vi "De-construct.vi"(10 "msg o":string) -> (0 "MSES/SRES":string, 1 "RSP?":bool, 2 "Data":string, 5 "CMD":T1, 7 "header":string)   [LabVIEW 2020, in "FINS TCP.lvlib"]
uses:
  FINS TCP.lvlib
  FINS CMD.ctl
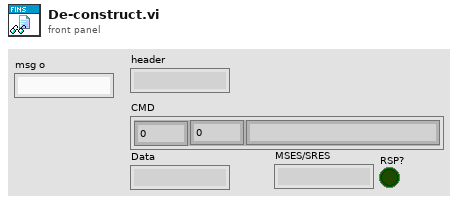
[diagram p1: front panel]
types:
  T1 = typedef "FINS TCP.lvlib/FINS CMD.ctl" = cluster{"MR":u8, "SR":u8, "name":string}
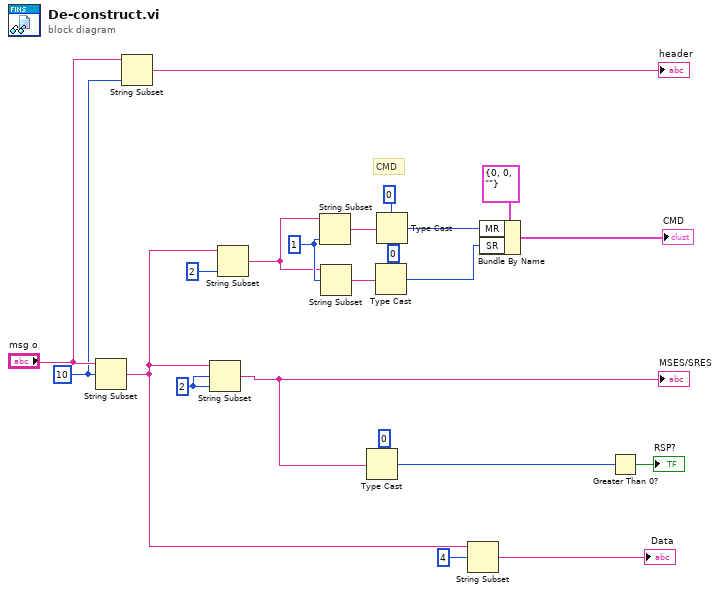
[diagram p0: block diagram]
diagram:
  w12 = 10 ("offset (0)")
  w21 = 1 ("length (rest)")
  w14 = 2 ("length (rest)")
  # "CMD"
  n1 = String Subset(string="msg o", offset (0)=w12) -> (substring=w15:string)  [unwired: 1 in]
  n2 = String Subset(string="msg o", length (rest)=w12) -> (substring=→"header":string)  [unwired: 1 in]
  n3 = String Subset(string=w15, offset (0)=w14, length (rest)=w14) -> (substring=w2:string)
  "MSES/SRES" <- w2
  n4 = String Subset(string=w15, length (rest)=2 ("length (rest)")) -> (substring=w16:string)  [unwired: 1 in]
  n5 = String Subset(string=w16, length (rest)=w21) -> (substring=w19:string)  [unwired: 1 in]
  n6 = String Subset(string=w16, offset (0)=w21) -> (substring=w20:string)  [unwired: 1 in]
  n7 = Type Cast(type=u16 0 ("length (rest)"), x=w2) -> (*(type *) &x=w1:u16)
  n8 = Type Cast(type=u8 0 ("length (rest)"), x=w20) -> (*(type *) &x=w9:u8)
  n9 = Type Cast(type=u8 0 ("length (rest)"), x=w19) -> (*(type *) &x=w10:u8)
  n10 = String Subset(string=w15, offset (0)=4 ("length (rest)")) -> (substring=→"Data":string)  [unwired: 1 in]
  n11 = Bundle By Name(cluster=T1 {"MR"=0, "SR"=0, "name"=""} ("FINS CMD"), "MR"=w10, "SR"=w9) -> (→"CMD":T1)
  n12 = Greater Than 0?(x=w1) -> (x > 0?=→"RSP?":bool)
